vi "Close.vi"(8 "error in (no error)":errorcluster, 11 "VISA resource in":refnum<visa-resource-name>) -> (0 "error out":errorcluster)   [LabVIEW 2020, in "Global FIA milliGAT.lvlib"]
doc: "Performs an instrument error query before terminating the software connection to the instrument."
uses:
  <instrlib>/RxnRover/Global FIA milliGAT 3.14/Global FIA milliGAT.lvlib
  <instrlib>/RxnRover/Global FIA milliGAT 3.14/Public/Utility/Pump Address.ctl
  <instrlib>/RxnRover/Global FIA milliGAT 3.14/Private/Pump Parameter.ctl
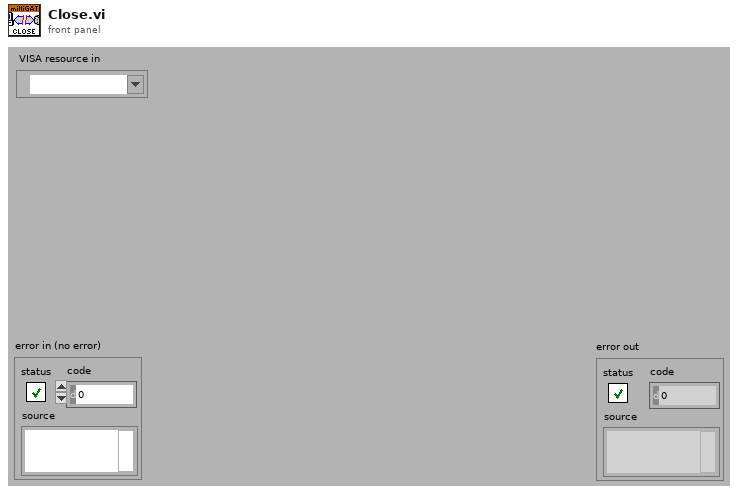
[diagram p1: front panel]
types:
  T1 = typedef "Global FIA milliGAT.lvlib/Pump Address.ctl" = enum16{"A", "B", "C", "D", "E", "F", "G", "H", "I", "J", "K", "L", "M", "N", "O", "P", "Q", "R", "S", "T", "U", "V", "W", "X", "Y", "Z", "a", "b", "c", "d", "e", "f", "g", "h", "i", "j", "k", "l", "m", "n", "o", "p", "q", "r", "s", "t", "u", "v", "w", "x", "y", "z", "0", "1", "2", "3", "4", "5", "6", "7", "8", "9"}
  T2 = typedef "Global FIA milliGAT.lvlib/Pump Parameter.ctl" = enum16{"Enabled", "EU", "EU Calibration Factor", "Fixed Asp or Disp", "Starting Position", "Starting Flow", "Peak Flow", "Flow Acceleration", "Flow Deceleration", "Session Volume", "Max Pressure", "Backlash (usteps)", "BL Calibration Factor", "BL Correction Enabled", "Min Flow", "Max Flow", "Min Acceleration", "Max Acceleration", "Service Volume", "Life Volume"}
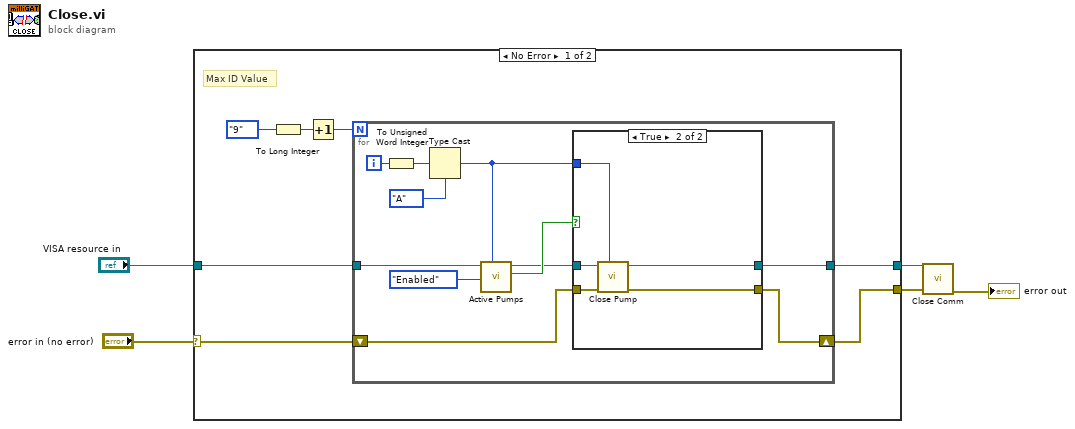
[diagram p0: block diagram]
diagram:
  n1 = case shown="No Error" "error in (no error)" {
    selector: "error in (no error)" -> [w6 w32]
    tunnel: "VISA resource in" -> [w9 w31]
    tunnel: [w8 w32] -> w2
    tunnel: [w7 w31] -> w3
    frame No Error {
      # "Max ID Value"
      n2 = To Long Integer(number=Pump_Address."9" ("Pump ID (0:A)")) -> (32bit integer=w10:i32)
      n3 = Increment(x=w10) -> (x+1=w11:i32)
      n4 = for {
        N: w11 -> [_]
        shift-right: [w18] -> w8
        shift-left: w6 -> [w19]
        tunnel: w9 -> [w14]
        tunnel: [w16] -> w7
        i -> [w23]
        n5 = To Unsigned Word Integer(number=w23) -> (unsigned 16bit integer=w20:u16)
        n6 = Type Cast(type=Pump_Address."A" ("Pump ID (0:A)"), x=w20) -> (*(type *) &x=w17:T1)
        n7 = call <instrlib>:"Active Pumps.vi"("Pump ID (0:A)"=w17, "Parameter"=Pump_Parameter."Enabled", "VISA resource in"=w14) -> ("Found"=w15:bool, "VISA resource out"=w13:refnum<visa-resource-name>)  [unwired: 5 in, 2 out]
        n8 = case shown="True" w15 {
          tunnel: w19 -> [w24 w29]
          tunnel: [w24 w26] -> w18
          tunnel: w13 -> [w25 w30]
          tunnel: w17 -> [_ w28]
          tunnel: [w25 w27] -> w16
          frame False {
            # "Pump never initialized"
          }
          frame True {
            n9 = call <instrlib>:"Close Pump.vi"("Pump ID (0:A)"=w28, "error in (no error)"=w29, "VISA resource in"=w30) -> ("error out"=w26:errorcluster, "VISA resource out"=w27:refnum<visa-resource-name>)  [unwired: 7 in]
          }
        }
      }
    }
    frame Error {
    }
  }
  n10 = call <instrlib>:"Close Comm.vi"("error in (no error)"=w2, "VISA resource in"=w3) -> ("error out"=→"error out":errorcluster)  [unwired: 9 in]
